vi "FindMissingIssues.vi"() -> ()   [LabVIEW 2024]
uses:
  <userlib>/_OpenG.lib/file/file.llb/Strip Path Extension - String__ogtk.vi
  <userlib>/_OpenG.lib/file/file.llb/openg_file.lvlib
panel:
  out "missing issues":i32[](array[numeric])
  in  "path":path
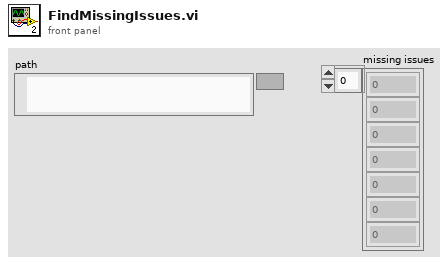
[diagram p1: front panel]
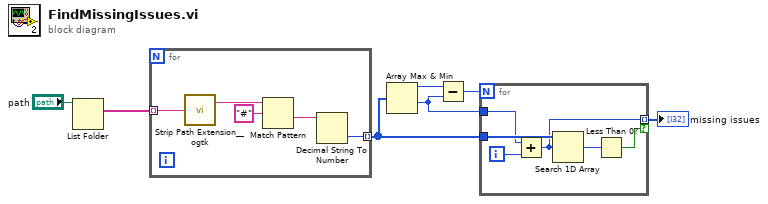
[diagram p0: block diagram]
diagram:
  n1 = List Folder(path="path") -> (filenames=w6:string[])  [unwired: 3 in, 3 out]
  n2 = for {
    tunnel: w6 -> [w12] mode=indexing
    tunnel: [w8] -> w4 mode=indexing
    n3 = call-poly <userlib>:"Strip Path Extension__ogtk.vi"("path"=w12) -> ("root"=w11:string)  [unwired: 1 out]
    n4 = Match Pattern(string=w11, regular expression="#") -> (after substring=w9:string)  [unwired: 1 in, 3 out]
    n5 = Decimal String To Number(string=w9) -> (number=w8:i32)  [unwired: 2 in, 1 out]
  }
  n6 = Array Max & Min(array=w4) -> (max value=w2:i32, min value=w1:i32)  [unwired: 2 out]
  n7 = Subtract(x=w2, y=w1) -> (x-y=w5:i32)
  n8 = for {
    N: w5 -> [_]
    tunnel: w4 -> [w18]
    tunnel: w1 -> [w16]
    tunnel: [w14] -> w3 mode=indexing if=w13
    i -> [w17]
    n9 = Add(x=w16, y=w17) -> (x+y=w14:i32)
    n10 = Search 1D Array(1D array=w18, element=w14) -> (index of element=w15:i32)  [unwired: 1 in]
    n11 = Less Than 0?(x=w15) -> (x < 0?=w13:bool)
  }
  "missing issues" <- w3
